vi "Dispenser.vi"() -> ()   [LabVIEW 2016]
uses:
  <vilib>/Utility/file.llb/Read Delimited Spreadsheet (string).vi
  Other Models/EFD Ultimus V/EFD Ultimus V.lvlib
panel:
  in  "Pressure":dbl[](array[numeric])=[27.0, 27.0, 27.0, 27.0]
  out "Time(ms)":dbl
  out "Speed":dbl format="%#_13g"
  out "Comm":string
  in  "VISA resource name":refnum<visa-resource-name>="COM5"
  in  "Serial Configuration":T1={"Baud Rate "=115200, "Parity "=0, "Data Bits "=8, "Stop Bits"=10} {"Stop Bits" items=["1.0"=10, "1.5"=15, "2.0"=20]; "Data Bits" items=["7"=7, "8"=8]; "Parity" items=["None", "Odd", "Even"]; "Baud Rate" items=["9600"=9600, "19200"=19200, "38400"=38400, "115200"=115200]}
  in  "Z":dbl=71.609 format="%#_13g"
  in  "Y":dbl=905.746 format="%#_13g"
  in  "X":dbl=435.404 format="%#_13g"
  in  "Path":path=path "C:/Users/TTUHEP/Documents/LabVIEW/Pattern/Modified_Standard_Pattern_2.ngc"
  # "Origin"
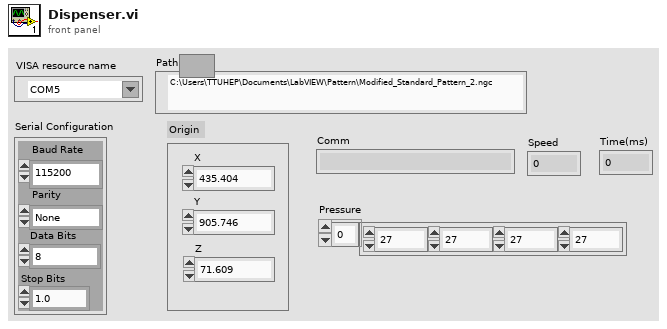
[diagram p1: front panel]
types:
  T1 = cluster{"Baud Rate ":u32, "Parity ":u16, "Data Bits ":u16, "Stop Bits":u16}
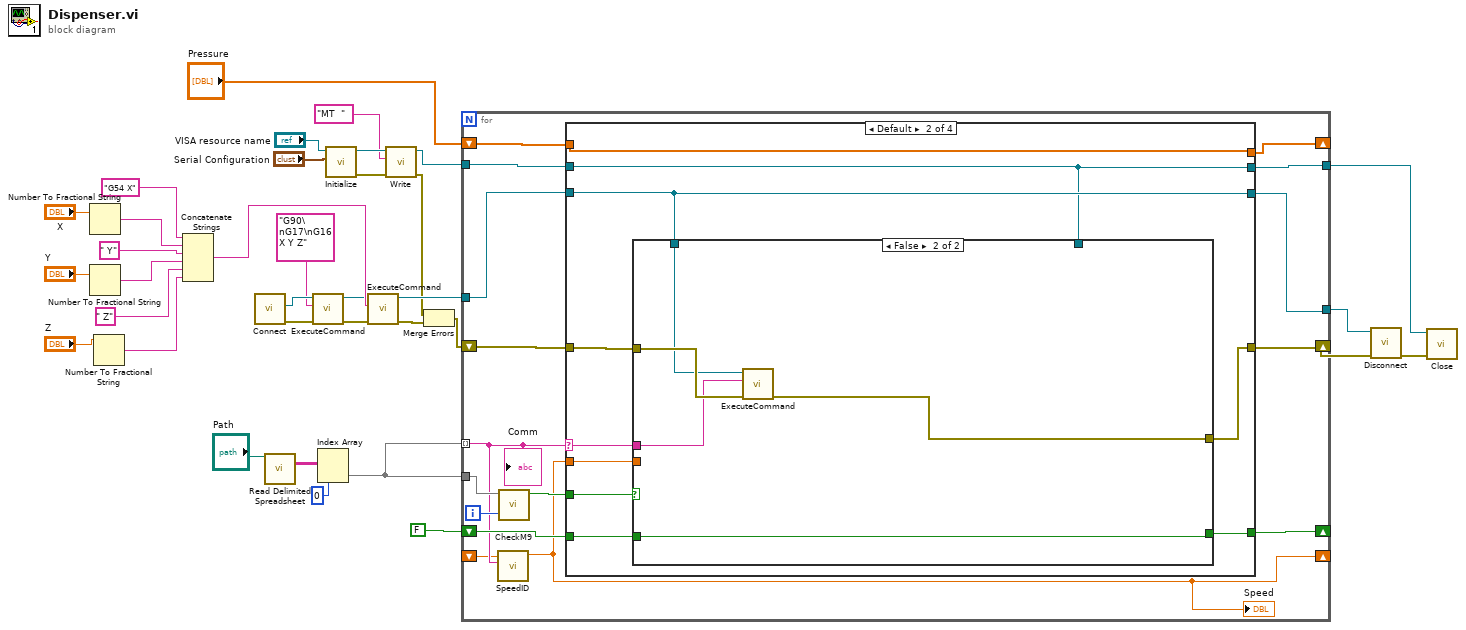
[diagram p0: block diagram]
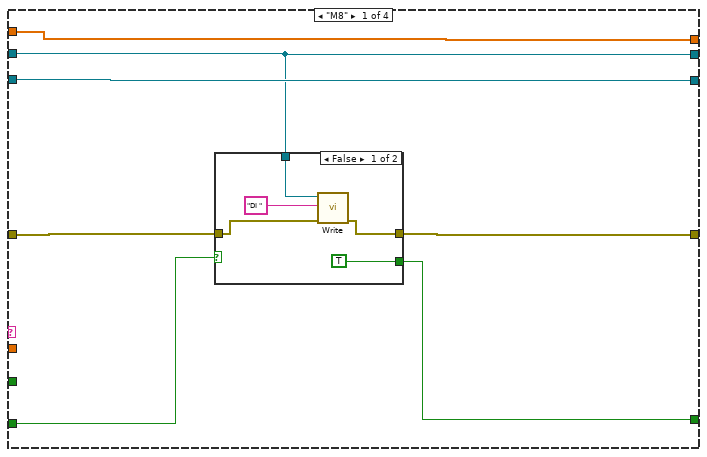
[diagram p2: hidden frame]
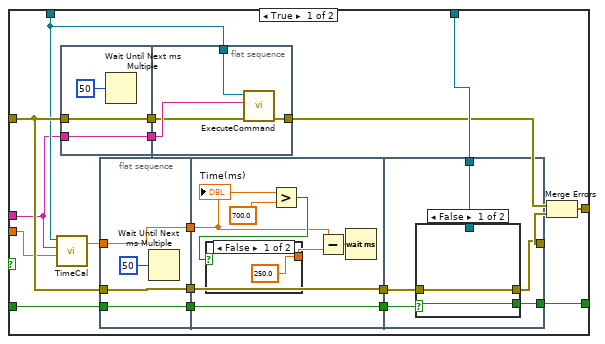
[diagram p4: hidden frame]
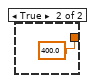
[diagram p5: hidden frame]
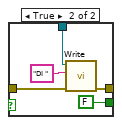
[diagram p6: hidden frame]
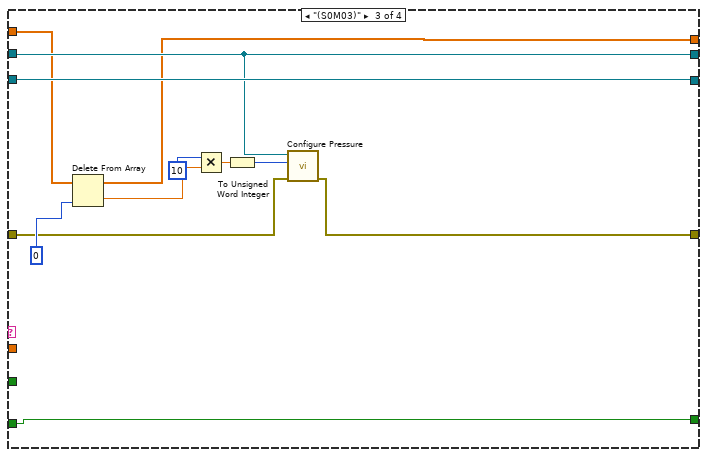
[diagram p7: hidden frame]
diagram:
  n1 = Number To Fractional String(number="X") -> (F-format string=w15:string)  [unwired: 3 in]
  n2 = Number To Fractional String(number="Y") -> (F-format string=w17:string)  [unwired: 3 in]
  n3 = Number To Fractional String(number="Z") -> (F-format string=w19:string)  [unwired: 3 in]
  n4 = Concatenate Strings("G54 X", w15, " Y", w17, " Z", w19) -> (w13:string)
  n5 = call "Connect.vi"() -> ("error out"=w2:errorcluster, "controller"=w12:refnum<k24>)  [unwired: 10 in]
  n6 = call-poly <vilib>:"Read Delimited Spreadsheet.vi"("file path (dialog if empty)"="Path") -> ("all rows"=w33:string[][])  [unwired: 9 in, 5 out]
  n7 = call "ExecuteCommand.vi"("Command Code"="G90\nG17\nG16 X Y Z", "controller in"=w12) -> ("controller out"=w3:refnum<k24>)  [unwired: 7 in, 2 out]
  n8 = Index Array(array=w33, index (col)=0) -> (element=w5:string[])  [unwired: 1 in]
  n9 = call "Initialize.vi"("Serial Configuration"="Serial Configuration", "VISA resource name"="VISA resource name") -> ("error out"=w9:errorcluster, "VISA resource name out"=w8:refnum<visa-resource-name>)  [unwired: 8 in]
  n10 = call "ExecuteCommand.vi"("error in (no error)"=w2, "Command Code"=w13, "controller in"=w3) -> ("error out"=w27:errorcluster, "controller out"=w30:refnum<k24>)  [unwired: 6 in, 1 out]
  n11 = call "Write.vi"("error in (no error)"=w9, "Command To Write"="MT  ", "VISA resource name"=w8) -> ("error out"=w6:errorcluster, "VISA resource name out"=w10:refnum<visa-resource-name>)  [unwired: 7 in]
  n12 = Merge Errors(w6, w27) -> (w26:errorcluster)
  n13 = for {
    tunnel: w5 -> [w40] mode=indexing
    shift-right: [w37] -> w25
    shift-left: w26 -> [w46]
    shift-right: [w48] -> _
    shift-left: FALSE -> [w49]
    tunnel: w30 -> [w47]
    tunnel: [w50] -> w4
    tunnel: w10 -> [w45]
    tunnel: [w44] -> w23
    tunnel: w5 -> [w43]
    shift-right: [w38] -> _
    shift-left: _ -> [w39]
    shift-right: [w35] -> _
    shift-left: "Pressure" -> [w36]
    i -> [w42]
    n14 = call "SpeedID.vi"("String"=w40, "Speed In"=w39) -> ("Speed Out"=w38:dbl)  [unwired: 9 in]
    "Speed" <- w38
    n15 = call "CheckM9.vi"("Index"=w42, "Comm list"=w43) -> ("Gonna Stop Next"=w41:bool)  [unwired: 9 in]
    n16 = case shown="Default" w40 {
      selector: w40 -> [_ w72 _ _]
      tunnel: w46 -> [w52 w74 w131 w145]
      tunnel: w47 -> [w57 w73 w141 w143]
      tunnel: [w56 w66 w130 w145] -> w37
      tunnel: [w57 w73 w141 w143] -> w50
      tunnel: w49 -> [w55 w70 w140 w146]
      tunnel: [w54 w69 w140 w146] -> w48
      tunnel: w45 -> [w53 w71 w139 w144]
      tunnel: [w53 w71 w139 w144] -> w44
      tunnel: w41 -> [_ w68 _ _]
      tunnel: w38 -> [_ w67 _ _]
      tunnel: w36 -> [w51 w65 w137 w142]
      tunnel: [w51 w65 w135 w142] -> w35
      frame "M8" {
        n17 = case shown="False" w55 {
          selector: w55 -> [_ w63]
          tunnel: w52 -> [w60 w64]
          tunnel: [w59 w64] -> w56
          tunnel: [TRUE w63] -> w54
          tunnel: w53 -> [w61 _]
          frame False {
            n18 = call "Write.vi"("error in (no error)"=w60, "Command To Write"="DI ", "VISA resource name"=w61) -> ("error out"=w59:errorcluster)  [unwired: 7 in, 1 out]
          }
          frame True {
          }
        }
      }
      frame Default {
        n19 = case shown="False" w68 {
          tunnel: w74 -> [w84 w129]
          tunnel: [w82 w128] -> w66
          tunnel: w73 -> [w77 w127]
          tunnel: w72 -> [w76 w126]
          tunnel: w71 -> [w90 _]
          tunnel: w70 -> [w92 w125]
          tunnel: [w91 w125] -> w69
          tunnel: w67 -> [w75 _]
          frame True {
            n20 = call "TimeCal.vi"("Speed In"=w75, "Command"=w76, "controller in"=w77) -> ("Time(ms)"=w78:dbl)  [unwired: 7 in, 1 out]
            n21 = flat-sequence {
              tunnel: w76 -> [w119]
              tunnel: [w119] -> w85
              tunnel: w84 -> [w118]
              tunnel: [w118] -> w83
              tunnel: w85 -> [w124]
              tunnel: w83 -> [w123]
              tunnel: [w122] -> w80
              tunnel: w77 -> [w121]
              frame #0 {
                n22 = Wait Until Next ms Multiple(millisecond multiple=50) -> ()  [unwired: 1 out]
              }
              frame #1 {
                n23 = call "ExecuteCommand.vi"("error in (no error)"=w123, "Command Code"=w124, "controller in"=w121) -> ("error out"=w122:errorcluster)  [unwired: 6 in, 2 out]
              }
            }
            n24 = flat-sequence {
              tunnel: w92 -> [w96]
              tunnel: [w96] -> w88
              tunnel: [w94] -> w87
              tunnel: w84 -> [w94]
              tunnel: w78 -> [w93]
              tunnel: [w93] -> w79
              tunnel: [w103] -> w89
              tunnel: w88 -> [w103]
              tunnel: w87 -> [w102]
              tunnel: [w102] -> w86
              tunnel: w79 -> [w97]
              tunnel: [w109] -> w91
              tunnel: [w108] -> w81
              tunnel: w90 -> [w107]
              tunnel: w89 -> [w110]
              tunnel: w86 -> [w106]
              frame #0 {
                n25 = Wait Until Next ms Multiple(millisecond multiple=50) -> ()  [unwired: 1 out]
              }
              frame #1 {
                n26 = Greater?(x=w97, y=700.0) -> (0:w99:bool)
                n27 = case shown="False" w99 {
                  tunnel: [250.0 400.0] -> w100
                  frame False {
                  }
                  frame True {
                  }
                }
                n28 = Subtract(x=w97, y=w100) -> (x-y=w101:dbl)
                n29 = Wait (ms)(milliseconds to wait=w101) -> ()  [unwired: 1 out]
                "Time(ms)" <- w97
              }
              frame #2 {
                n30 = case shown="False" w110 {
                  selector: w110 -> [w111 _]
                  tunnel: w106 -> [w112 w116]
                  tunnel: [w112 w115] -> w108
                  tunnel: [w111 FALSE] -> w109
                  tunnel: w107 -> [_ w114]
                  frame False {
                  }
                  frame True {
                    n31 = call "Write.vi"("error in (no error)"=w116, "Command To Write"="DI ", "VISA resource name"=w114) -> ("error out"=w115:errorcluster)  [unwired: 7 in, 1 out]
                  }
                }
              }
            }
            n32 = Merge Errors(w80, w81) -> (w82:errorcluster)
          }
          frame False {
            n33 = call "ExecuteCommand.vi"("error in (no error)"=w129, "Command Code"=w126, "controller in"=w127) -> ("error out"=w128:errorcluster)  [unwired: 6 in, 2 out]
          }
        }
      }
      frame "(S0M03)" {
        n34 = Delete From Array(array=w137, index=0) -> (deleted portion=w134:dbl, array with subset deleted=w135:dbl[])  [unwired: 1 in]
        n35 = Multiply(x=10, y=w134) -> (x*y=w133:dbl)
        n36 = To Unsigned Word Integer(number=w133) -> (unsigned 16bit integer=w132:u16)
        n37 = call "Configure Pressure.vi"("error in (no error)"=w131, "Pressure Setting (0000)"=w132, "VISA resource name"=w139) -> ("error out"=w130:errorcluster)  [unwired: 7 in, 1 out]
      }
      frame "M9" {
      }
    }
    "Comm" <- w40
  }
  n38 = call "Disconnect.vi"("error in (no error)"=w25, "controller"=w4) -> ("error out"=w24:errorcluster)  [unwired: 9 in]
  n39 = call "Close.vi"("error in (no error)"=w24, "VISA resource name"=w23) -> ()  [unwired: 9 in, 1 out]
